vi "曲线记录.vi"(8 "文件名":string, 9 "检测序号":string="00000", 11 "波形图表in":refnum<vi>) -> ()   [LabVIEW 2018]
uses:
  <vilib>/Utility/file.llb/Write Delimited Spreadsheet (DBL).vi
panel:
  out "大小":i32
  out "路径":path
  in  "时间标识":timestamp
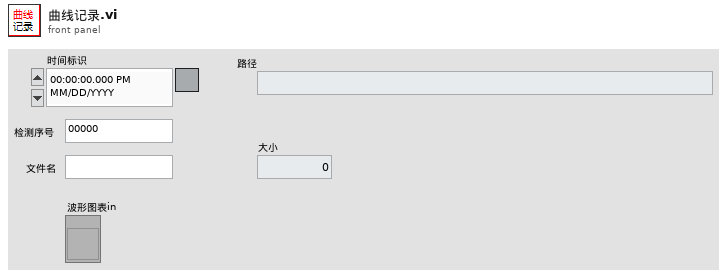
[diagram p1: front panel]
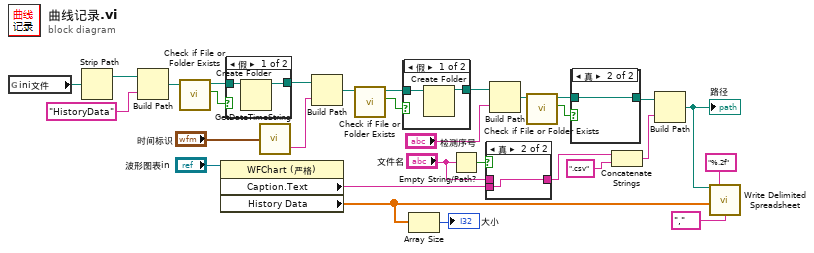
[diagram p0: block diagram]
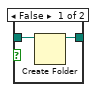
[diagram p4: hidden frame]
diagram:
  n1 = global read "全局 1.vi" "ini文件"() -> (w30:path)
  n2 = Strip Path(path=w30) -> (stripped path=w29:path)  [unwired: 1 out]
  n3 = Build Path(base path=w29, name or relative path="HistoryData" ("名称或相对路径")) -> (appended path=w4:path)
  n4 = call <vilib>:"Check if File or Folder Exists.vi"("path"=w4) -> ("file or folder exists?"=w2:bool, "dup path"=w3:path)  [unwired: 8 in, 1 out]
  n5 = property class="WFChart (严格)"(reference="波形图表in") -> ("Caption.Text"=w13:string, "History Data"=w6:dbl[])  [unwired: 1 in, 2 out]
  n6 = case shown="假" w2 {
    tunnel: w3 -> [w32 w33]
    tunnel: [w31 w33] -> w1
    frame False {
      n7 = Create Folder(path (use dialog)=w32) -> (created path=w31:path)  [unwired: 2 in, 2 out]
    }
    frame True {
    }
  }
  n8 = call "GetDateTimeString.vi"("time stamp"="时间标识") -> ("YYYYMMDD"=w26:string)  [unwired: 3 in, 1 out]
  n9 = Build Path(base path=w1, name or relative path=w26) -> (appended path=w25:path)
  n10 = call <vilib>:"Check if File or Folder Exists.vi"("path"=w25) -> ("file or folder exists?"=w24:bool, "dup path"=w23:path)  [unwired: 8 in, 1 out]
  n11 = case shown="假" w24 {
    tunnel: w23 -> [w35 w36]
    tunnel: [w34 w36] -> w22
    frame False {
      n12 = Create Folder(path (use dialog)=w35) -> (created path=w34:path)  [unwired: 2 in, 2 out]
    }
    frame True {
    }
  }
  n13 = Array Size(array=w6) -> (size(s)=→"大小":i32)
  n14 = Empty String/Path?(string/path="文件名") -> (empty?=w11:bool)
  n15 = case shown="真" w11 {
    tunnel: w13 -> [_ w38]
    tunnel: "文件名" -> [w37 _]
    tunnel: [w37 w38] -> w9
    frame False {
    }
    frame True {
    }
  }
  n16 = Build Path(base path=w22, name or relative path="检测序号") -> (appended path=w21:path)
  n17 = call <vilib>:"Check if File or Folder Exists.vi"("path"=w21) -> ("file or folder exists?"=w20:bool, "dup path"=w19:path)  [unwired: 8 in, 1 out]
  n18 = case shown="真" w20 {
    tunnel: w19 -> [w40 w41]
    tunnel: [w39 w41] -> w18
    frame False {
      n19 = Create Folder(path (use dialog)=w40) -> (created path=w39:path)  [unwired: 2 in, 2 out]
    }
    frame True {
    }
  }
  n20 = Concatenate Strings(w9, ".csv" ("字符串")) -> (w8:string)
  n21 = Build Path(base path=w18, name or relative path=w8) -> (appended path=w14:path)
  "路径" <- w14
  n22 = call-poly <vilib>:"Write Delimited Spreadsheet.vi"("file path (dialog if empty)"=w14, "format (%.3f)"="%.2f", "1D data"=w6, "delimiter (\\t)"="," ("delimiter (\\t)")) -> ()  [unwired: 10 in, 2 out]
